vi "CAN_MotorControlandBMS2.vi"() -> ()   [LabVIEW 2018]
uses:
  BMS/OrionBMSClass.lvclass
  <vilib>/Platform/TimedLoop/XDataNode/wakeup.ctl
  <vilib>/Platform/TimedLoop/XDataNode/XDNodeRunTimeDep.lvlib
  <vilib>/Platform/TimedLoop/XDataNode/nitl_modes.ctl
  <vilib>/Platform/TimedLoop/XDataNode/timing_clust.ctl
  <vilib>/platform/TimedLoop/XDataNode/XDataNode.xnode
  Type_Def/Type_Def MotorControlState.ctl
  BMS/MotorControllerClass.lvclass
  Type_Def/TypeDef_MotorData.ctl
  <vilib>/Platform/TimedLoop/XDataNode/loadnilvce.vi
  Type_Def/TypeDef_BMSDatas.ctl
  Type_Def/TypeDef_BMSStatuss.ctl
  Type_Def/Type_Def Actuator Controls.ctl
panel:
  out "BMS2 Freeze":bool
  in  "ReintCAN":bool
  in  "GlobalStop":bool
  in  "Reset BMS Freeze":bool
  in  "stop":bool
  out "Velocity (RPM)":i32
  out "error out":errorcluster
  out "Loop Counter":i32
  out "BMS1 Freeze":bool
  out "stopDriveRes":u32
  out "changeTargetRes":u32
  out "targetTorqueRes":u32
  out "controlWord6Res":i16
  out "startDriveRes":u32
  out "Enum":T1
  in  "error in (no error)":errorcluster
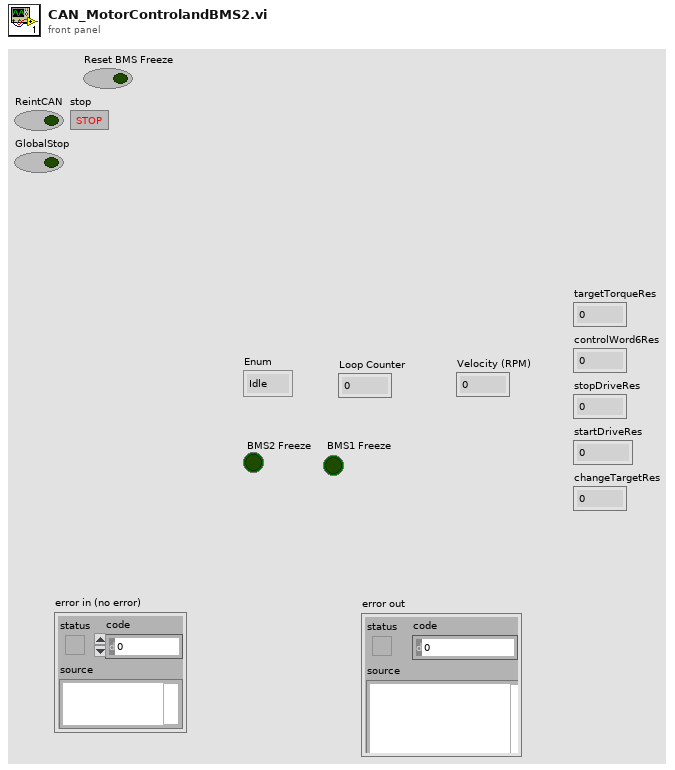
[diagram p1: front panel]
types:
  T1 = typedef "Type_Def MotorControlState.ctl" = enum16{"Idle", "Initialization", "Running", "Termination"}
  T2 = enum32{"1 Mbit/s", "800 kbit/s", "500 kbit/s", "250 kbit/s", "125 kbit/s", "50 kbit/s", "20 kbit/s", "10 kbit/s", ""}
  T3 = typedef "TypeDef_MotorData.ctl" = cluster{" Velocity (RPM)":i32, " MotorTemp(C)":u8, " ControlTemp(C)":u8, " DcLinkVolt(V)":dbl, " ErrorCode":dbl, "IsAlive":bool, "motorStatus":cluster{"isReady":bool, "isOn":bool, "isOperEn":bool, "isFault":bool, "isVoltEn":bool, "targetReached":bool, "isWarning":bool}, "motorControllerState":u16}
  T4 = typedef "XDNodeRunTimeDep.lvlib/timing_clust.ctl" = cluster{"Expected End [f-1]":u64, "Actual End [f-1]":u64, "Finished Late? [f-1]":bool, "Expected End [i-1]":u64, "Actual End [i-1]":u64, "Finished Late? [i-1]":bool, "Expected Start [i]":u64, "Actual Start [i]":u64, "Expected Start [f]":u64, "Actual Start [f]":u64, "Source Name":string, "Structure Name":string, "Period":i64, "Deadline":i64, "Offset":i64, "Start":i64, "Priority":i32, "Timeout":i32, "Mode":T5, "Wakeup Reason":T6, "Error":errorcluster, "Source Type":string, "Secondary Source Type":string, "Global End Time":u64, "Global Start Time":u64, "Frame Duration":u64, "Iteration Duration":u64, "Assigned CPU":i32, "I/O Scan Engine Mode":u32}
  T5 = typedef "XDNodeRunTimeDep.lvlib/nitl_modes.ctl" = enum32{"No Change", "Process missed periods, maintain original phase", "Discard missed periods, maintain original phase", "Process missed periods, ignore original phase", "Discard missed periods, ignore original phase"}
  T6 = typedef "XDNodeRunTimeDep.lvlib/wakeup.ctl" = enum32{"Normal", "Aborted", "Asynchronous wakeup", "Timing source error", "Timed loop error", "Timeout"}
  T7 = typedef "Type_Def Actuator Controls.ctl" = cluster{"Reverse ":bool, "Precharge Ctrl":bool, "Pump Ctrl":bool, "24 VDC Ctr":bool, "Vent Solenoid":bool, "Brake Solenoid":bool, "EMCY  Brake Solenoid":bool, "Digital Out 7B ":bool, "Forward Ctrl":bool, " Contact H2":bool, "Contact L2":bool, "LED RED":bool, "LED GREEN":bool, " Digital Out 7A":bool, " Contact H1":bool, "Contact L1":bool}
  T8 = typedef "TypeDef_BMSDatas.ctl" = cluster{"Pack 1 Max Cell\n Voltage (V)":dbl, "Pack 1 Max Cell\n ID ":dbl, "Pack 1 Min Cell \nVoltage (V)":dbl, "Pack 1 Min Cell \nID ":dbl, "Pack 1 State of Charge  (%)":dbl, "Pack 1 Average Voltage1 (V)":dbl, "Pack 1Voltage Delta (V)":dbl, "Pack 1 Current (A)":dbl, "Pack 1 Voltage (V)":dbl, "Pack 1 Max Resistance (Ohm)":dbl, "Pack 1Min Resistance (Ohm)":dbl, "Pack 1Average Resistance (Ohm)":dbl, "Pack 1Delta Resistance (Ohm)":dbl, "Pack 1 Highest Temperature(C)":dbl, "BmsStatus1":T9, "Pack 2 Max Cell\n Voltage (V) ":dbl, "Pack 2 Max Cell\n ID  ":dbl, "Pack 2 Min Cell \nVoltage (V) ":dbl, "Pack 2 Min Cell \nID  ":dbl, "Pack 2 Average Voltage1 (V)":dbl, "Pack 2 Voltage Delta (V) ":dbl, "Pack 2 Current (A)":dbl, "Pack 2 Voltage (V) ":dbl, "Pack 2 State of Charge  (%) ":dbl, "Pack 2 Max Resistance (Ohm) ":dbl, "Pack 2 Min Resistance (Ohm)":dbl, "Pack 2 Average Resistance (Ohm)":dbl, "Pack 2 Delta Resistance (Ohm) ":dbl, "Pack 2 Highest Temperature(C) ":dbl, "BmsStatus 2":T9}
  T9 = typedef "TypeDef_BMSStatuss.ctl" = cluster{"isFault":bool, "isolationMonitoring":bool}
  T10 = cluster{"error code":dbl, "error register":dbl, "manufacturer specific error field":dbl[]}
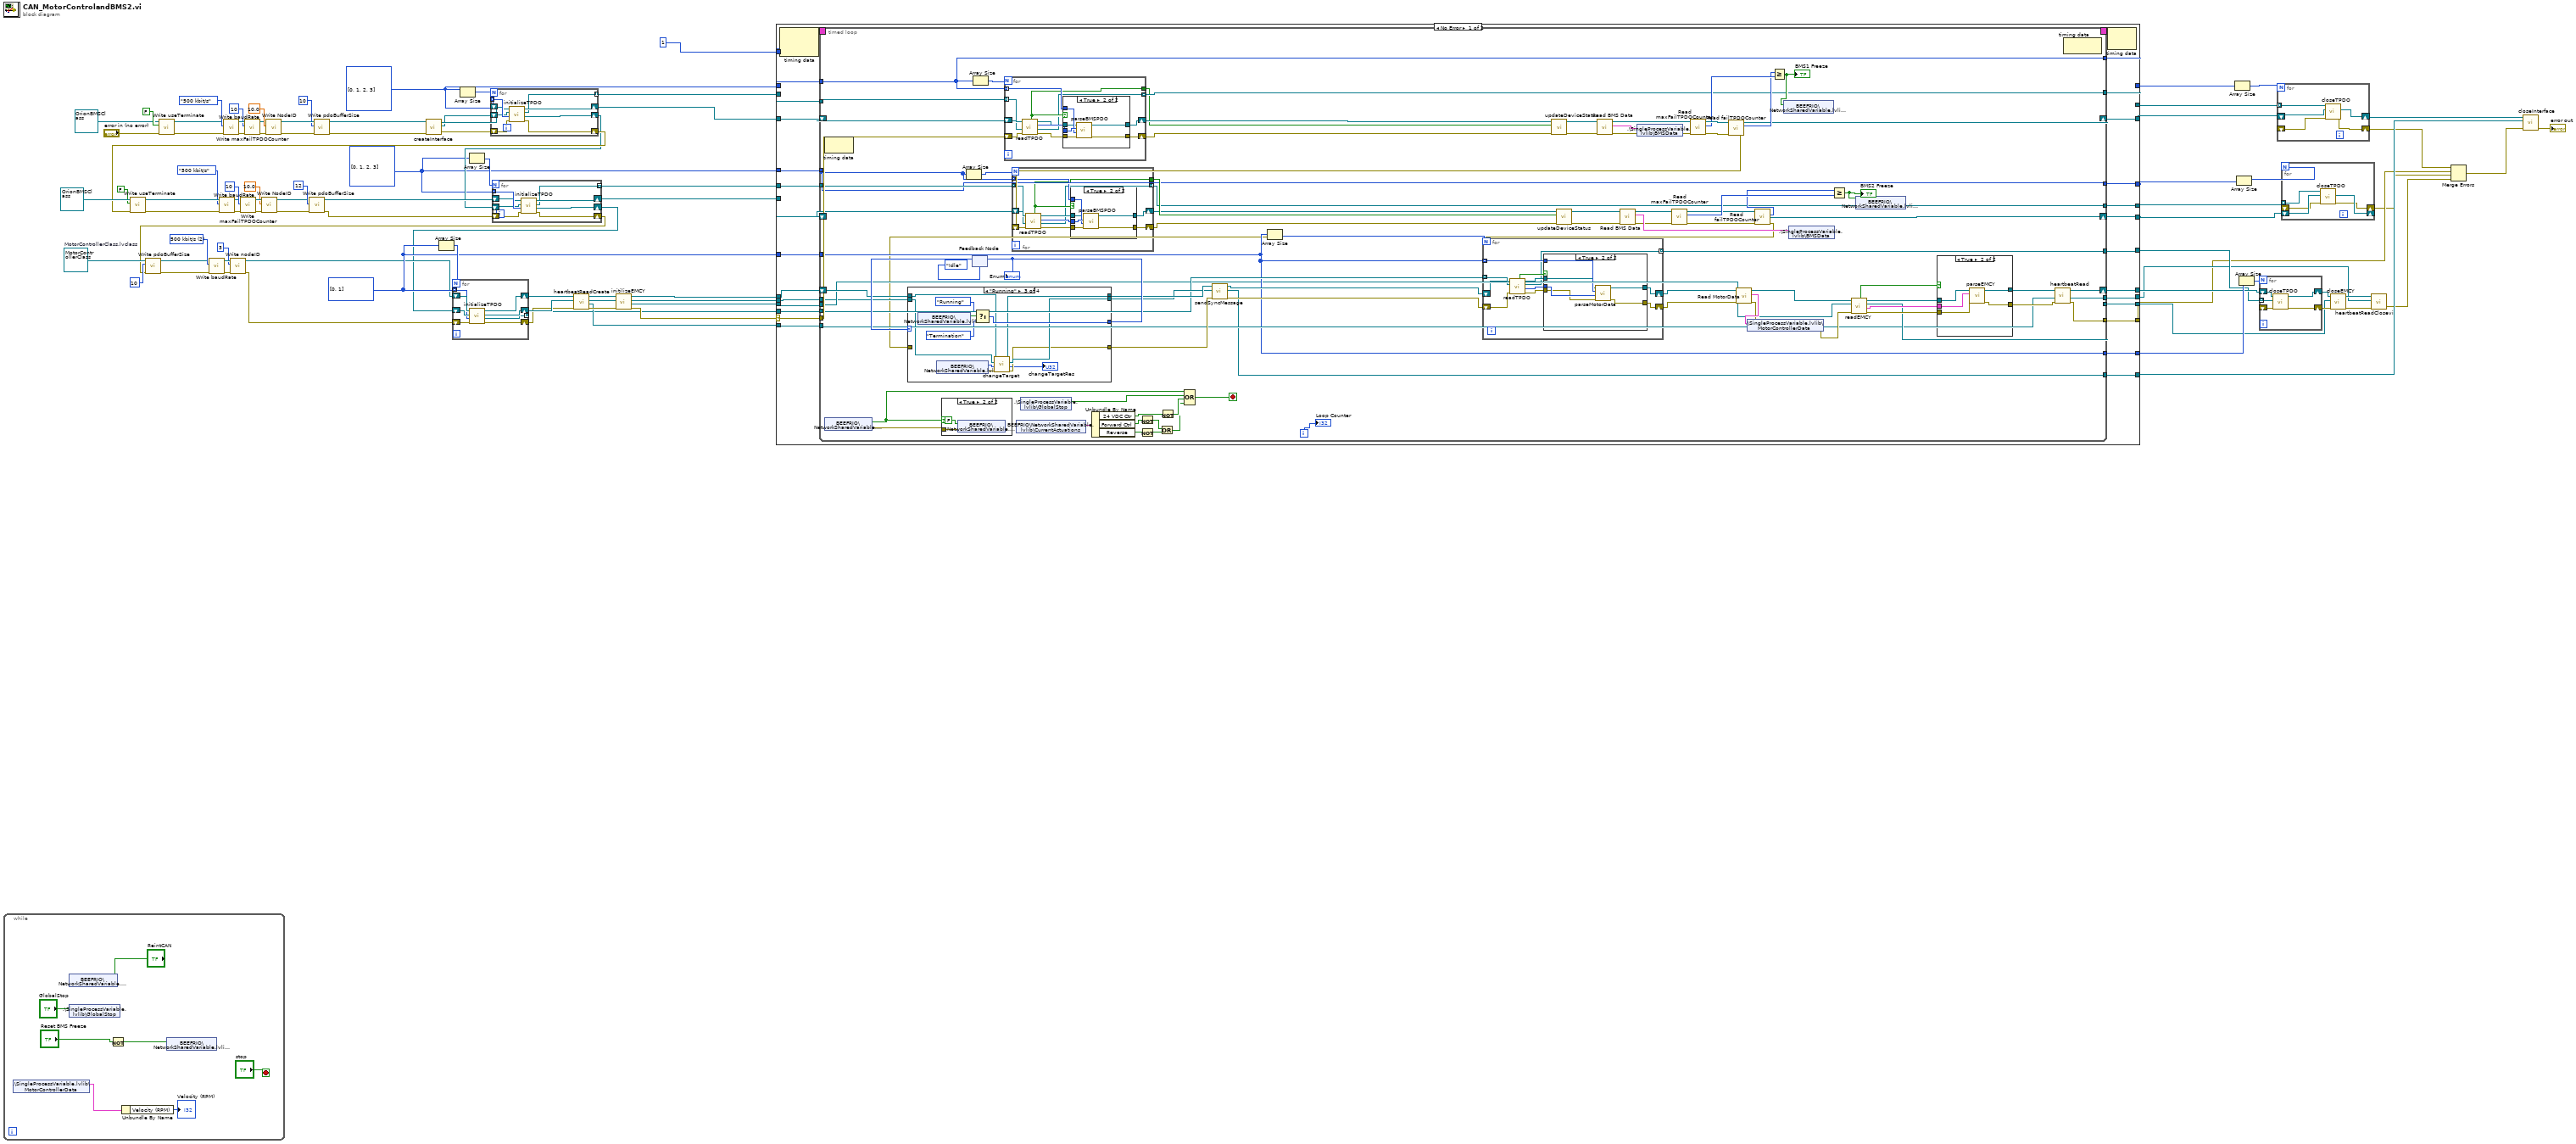
[diagram p0: block diagram]
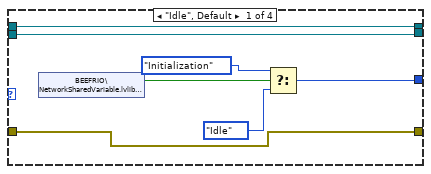
[diagram p6: hidden frame]
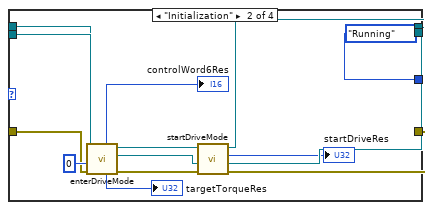
[diagram p7: hidden frame]
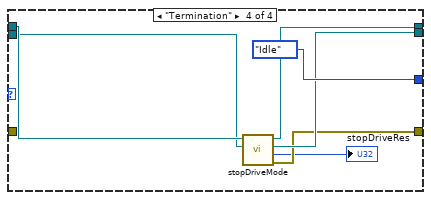
[diagram p8: hidden frame]
diagram:
  w8 = u8[] [0, 1, 2, 3] items=["PDO 1", "PDO 2", "PDO 3", "PDO 4"]
  w46 = u32 2 items=["1 Mbit/s"=0, "800 kbit/s"=1, "500 kbit/s"=2, "250 kbit/s"=3, "125 kbit/s"=4, "50 kbit/s"=6, "20 kbit/s"=7, "10 kbit/s"=8] ("baudRate")
  w78 = u8[] [0, 1] items=["PDO 1", "PDO 2", "PDO 3", "PDO 4"]
  w50 = refnum<class "MotorControllerClass.lvclass"> refnum  # MotorControllerClass.lvclass
  w10 = u8[] [0, 1, 2, 3] items=["PDO 1", "PDO 2", "PDO 3", "PDO 4"]
  n1 = while {
    stop <- "stop" stop-if-true
    n2 = shared-variable ".\\SingleProcessVariable.lvlib\\MotorControllerData"() -> (w101:T3)  [unwired: 1 in, 1 out]
    n3 = shared-variable "BEEFRIO\\NetworkSharedVariable.lvlib\\ReintCAN"("ReintCAN") -> ()  [unwired: 1 in, 1 out]
    n4 = shared-variable ".\\SingleProcessVariable.lvlib\\GlobalStop"("GlobalStop") -> ()  [unwired: 1 in, 1 out]
    n5 = Not(x="Reset BMS Freeze") -> (.not. x?=w103:bool)
    n6 = Unbundle By Name(w101) -> ("Velocity (RPM)"=→"Velocity (RPM)":i32)
    n7 = shared-variable "BEEFRIO\\NetworkSharedVariable.lvlib\\BMSFreeze"(w103) -> ()  [unwired: 1 in, 1 out]
  }
  n8 = call-dynamic "Write useTerminate .vi"("error in (no error)"="error in (no error)", "useTerminate"=FALSE, "OrionBMS in"=refnum<class "OrionBMSClass.lvclass"> refnum ("OrionBMSClass.lvclass")) -> ("error out"=w36:errorcluster, "OrionBMS out"=w37:refnum<class "OrionBMSClass.lvclass">)  [unwired: 7 in]
  n9 = call-dynamic "Write baudRate.vi"("error in (no error)"=w36, "baudRate"=T2."500 kbit/s", "OrionBMSClass in"=w37) -> ("error out"=w42:errorcluster, "OrionBMSClass out"=w43:refnum<class "OrionBMSClass.lvclass">)  [unwired: 7 in]
  n10 = call-dynamic "Write maxFailTPDOCounter.vi"("error in (no error)"=w42, "maxFailTPDOCounter"=u8 10, "OrionBMSClass in"=w43) -> ("error out"=w40:errorcluster, "OrionBMSClass out"=w41:refnum<class "OrionBMSClass.lvclass">)  [unwired: 7 in]
  n11 = call-dynamic "Write NodeID.vi"("error in (no error)"=w40, "NodeID"=10.0, "OrionBMSClass in"=w41) -> ("error out"=w58:errorcluster, "OrionBMSClass out"=w59:refnum<class "OrionBMSClass.lvclass">)  [unwired: 7 in]
  n12 = call-dynamic "Write pdoBufferSize.vi"("error in (no error)"=w58, "pdoBufferSize"=u16 10, "OrionBMSClass in"=w59) -> ("error out"=w56:errorcluster, "OrionBMSClass out"=w57:refnum<class "OrionBMSClass.lvclass">)  [unwired: 7 in]
  n13 = call "createInterface.vi"("error in (no error)"=w56, "OrionBMS in"=w57) -> ("error out"=w95:errorcluster, "interface object out"=w96:refnum<k20>, "OrionBMS out"=w97:refnum<class "OrionBMSClass.lvclass">)  [unwired: 7 in]
  n14 = Array Size(array=w78) -> (size(s)=w89:i32)
  n15 = Array Size(array=w10) -> (size(s)=w11:i32)
  n16 = Array Size(array=w8) -> (size(s)=w9:i32)
  n17 = for {
    N: w11 -> [_]
    tunnel: w10 -> [w114] mode=indexing
    shift-right: [w110] -> w94
    shift-left: w97 -> [w113]
    tunnel: [w107] -> w93 mode=indexing
    shift-right: [w109] -> w12
    shift-left: w96 -> [w112]
    shift-right: [w108] -> w16
    shift-left: w95 -> [w111]
    n18 = call "initializeTPDO.vi"("error in (no error)"=w111, "PDO channel"=w114, "interface object in"=w112, "OrionBMS in"=w113) -> ("error out"=w108:errorcluster, "interface object out"=w109:refnum<k20>, "TPDO object out"=w107:refnum<k20>, "OrionBMS out"=w110:refnum<class "OrionBMSClass.lvclass">)  [unwired: 2 in]
  }
  n19 = call-dynamic "Write useTerminate .vi"("error in (no error)"=w16, "useTerminate"=FALSE, "OrionBMS in"=refnum<class "OrionBMSClass.lvclass"> refnum ("OrionBMSClass.lvclass")) -> ("error out"=w32:errorcluster, "OrionBMS out"=w31:refnum<class "OrionBMSClass.lvclass">)  [unwired: 7 in]
  n20 = call-dynamic "Write baudRate.vi"("error in (no error)"=w32, "baudRate"=T2."500 kbit/s", "OrionBMSClass in"=w31) -> ("error out"=w27:errorcluster, "OrionBMSClass out"=w26:refnum<class "OrionBMSClass.lvclass">)  [unwired: 7 in]
  n21 = call-dynamic "Write maxFailTPDOCounter.vi"("error in (no error)"=w27, "maxFailTPDOCounter"=u8 10, "OrionBMSClass in"=w26) -> ("error out"=w29:errorcluster, "OrionBMSClass out"=w28:refnum<class "OrionBMSClass.lvclass">)  [unwired: 7 in]
  n22 = call-dynamic "Write NodeID.vi"("error in (no error)"=w29, "NodeID"=10.0, "OrionBMSClass in"=w28) -> ("error out"=w22:errorcluster, "OrionBMSClass out"=w21:refnum<class "OrionBMSClass.lvclass">)  [unwired: 7 in]
  n23 = call-dynamic "Write pdoBufferSize.vi"("error in (no error)"=w22, "pdoBufferSize"=u16 12, "OrionBMSClass in"=w21) -> ("error out"=w19:errorcluster, "OrionBMSClass out"=w18:refnum<class "OrionBMSClass.lvclass">)  [unwired: 7 in]
  n24 = for {
    N: w9 -> [_]
    tunnel: w8 -> [w122] mode=indexing
    shift-right: [w118] -> w13
    shift-left: w18 -> [w121]
    tunnel: [w115] -> w14 mode=indexing
    shift-right: [w117] -> w1
    shift-left: w12 -> [w120]
    shift-right: [w116] -> w15
    shift-left: w19 -> [w119]
    n25 = call "initializeTPDO.vi"("error in (no error)"=w119, "PDO channel"=w122, "interface object in"=w120, "OrionBMS in"=w121) -> ("error out"=w116:errorcluster, "interface object out"=w117:refnum<k20>, "TPDO object out"=w115:refnum<k20>, "OrionBMS out"=w118:refnum<class "OrionBMSClass.lvclass">)  [unwired: 2 in]
  }
  n26 = call-dynamic "Write pdoBufferSize.vi"("error in (no error)"=w15, "pdoBufferSize"=u16 10, "MotorControllerClass in"=w50) -> ("error out"=w33:errorcluster, "MotorControllerClass out"=w34:refnum<class "MotorControllerClass.lvclass">)  [unwired: 7 in]
  n27 = call-dynamic "Write baudRate.vi"("error in (no error)"=w33, "baudRate"=w46, "MotorControllerClass in"=w34) -> ("error out"=w49:errorcluster, "MotorControllerClass out"=w52:refnum<class "MotorControllerClass.lvclass">)  [unwired: 7 in]
  n28 = call-dynamic "Write nodeID.vi"("error in (no error)"=w49, "nodeID"=u8 3, "MotorControllerClass in"=w52) -> ("error out"=w48:errorcluster, "MotorControllerClass out"=w51:refnum<class "MotorControllerClass.lvclass">)  [unwired: 7 in]
  n29 = for {
    N: w89 -> [_]
    tunnel: w78 -> [w128] mode=indexing
    tunnel: [w125] -> w77 mode=indexing
    shift-right: [w127] -> w88
    shift-left: w51 -> [w130]
    shift-right: [w126] -> w87
    shift-left: w1 -> [w129]
    shift-right: [w124] -> w86
    shift-left: w48 -> [w123]
    n30 = call "initializeTPDO.vi"("error in (no error)"=w123, "PDO channel"=w128, "interface object in"=w129, "MotorControllerClass in"=w130) -> ("error out"=w124:errorcluster, "TPDO object out"=w125:refnum<k20>, "interface object out"=w126:refnum<k20>, "MotorControllerClass out"=w127:refnum<class "MotorControllerClass.lvclass">)  [unwired: 4 in]
  }
  n31 = call "heartbeatReadCreate.vi"("error in (no error)"=w86, "interface object in"=w87, "MotorControllerClass in"=w88) -> ("error out"=w83:errorcluster, "heartbeat object out"=w82:refnum<k20>, "interface object out"=w84:refnum<k20>, "MotorControllerClass out"=w85:refnum<class "MotorControllerClass.lvclass">)  [unwired: 5 in]
  n32 = call "initilizeEMCY.vi"("error in (no error)"=w83, "interface object in"=w84, "MotorControllerClass in"=w85) -> ("error out"=w81:errorcluster, "emergency object out"=w35:refnum<k20>, "interface object out"=w79:refnum<k20>, "MotorControllerClass out"=w80:refnum<class "MotorControllerClass.lvclass">)  [unwired: 5 in]
  n33 = case shown="No Error" w81 {
    selector: w81 -> [w141 w369]
    tunnel: w10 -> [w157 w372]
    tunnel: w94 -> [w156 w371]
    tunnel: w93 -> [w155 w364]
    tunnel: [w132 w372] -> w75
    tunnel: [w151 w364] -> w38
    tunnel: w82 -> [w154 w366]
    tunnel: w80 -> [w142 w367]
    tunnel: w79 -> [w140 w365]
    tunnel: w78 -> [w153 w370]
    tunnel: w77 -> [w152 w368]
    tunnel: [w131 w371] -> w74
    tunnel: [w150 w366] -> w64
    tunnel: [w144 w363] -> w67
    tunnel: [w149 w369] -> w61
    tunnel: [w148 w370] -> w73
    tunnel: [w147 w367] -> w71
    tunnel: [w145 w368] -> w70
    tunnel: [w146 w365] -> w63
    tunnel: i64 1 ("Period") -> [w143 _]
    tunnel: w35 -> [w139 w363]
    tunnel: w14 -> [w138 w361]
    tunnel: w13 -> [w136 w360]
    tunnel: w8 -> [w137 w362]
    tunnel: [w135 w360] -> w5
    tunnel: [w134 w361] -> w6
    tunnel: [w133 w362] -> w4
    frame No Error {
      n34 = node-c288(w143) -> (w159:T4)  [unwired: 1 in]
      n35 = timed-loop {
        timing: w159 -> [_]
        timing-out: [_] -> w158
        tunnel: w157 -> [w230]
        tunnel: w155 -> [w244]
        tunnel: [w230] -> w132
        tunnel: [w229] -> w151
        tunnel: w154 -> [w204]
        tunnel: w153 -> [w201]
        tunnel: w152 -> [w220]
        tunnel: [w207] -> w144
        tunnel: [w203] -> w149
        tunnel: [w202] -> w150
        tunnel: [w201] -> w148
        shift-right: [w200] -> w147
        shift-left: w142 -> [w225]
        tunnel: [w199] -> w145
        tunnel: [w198] -> w146
        tunnel: w139 -> [w187]
        tunnel: w141 -> [w226]
        tunnel: w140 -> [w185]
        shift-right: [w184] -> w131
        shift-left: w156 -> [w245]
        tunnel: w138 -> [w182]
        tunnel: w137 -> [w167]
        tunnel: [w167] -> w133
        tunnel: [w166] -> w134
        shift-right: [w165] -> w135
        shift-left: w136 -> [w163]
        i -> [w247]
        stop <- w161 stop-if-true
        n36 = node-c288() -> ()  [unwired: 1 in, 1 out]
        n37 = shared-variable "BEEFRIO\\NetworkSharedVariable.lvlib\\ReintCAN"() -> (w160:bool, error out=w193:errorcluster)  [unwired: 1 in]
        n38 = case shown="True" w160 {
          tunnel: w193 -> [_ w268]
          frame False {
          }
          frame True {
            n39 = shared-variable "BEEFRIO\\NetworkSharedVariable.lvlib\\ReintCAN"(FALSE ("ReintCAN"), error in=w268) -> ()  [unwired: 1 out]
          }
        }
        n40 = Array Size(array=w167) -> (size(s)=w183:i32)
        n41 = feedback #1(Type_Def_MotorControlState."Idle" ("Enum")) -> (w227:T1)
        n42 = Array Size(array=w230) -> (size(s)=w246:i32)
        n43 = for {
          N: w246 -> [_]
          tunnel: w244 -> [w344] mode=indexing
          tunnel: w230 -> [w341] mode=indexing
          tunnel: [w339] -> w162
          shift-right: [w338] -> w243
          shift-left: w245 -> [w345]
          shift-right: [w336] -> w242
          shift-left: w226 -> [w337]
          tunnel: [w335] -> w229 mode=indexing
          n44 = call "readTPDO.vi"("OrionBMS.lvclass"=w345, "TPDO object in"=w344, "error in (no error)"=w337) -> ("new data?"=w339:bool, "OrionBMS.lvclass"=w340:refnum<class "OrionBMSClass.lvclass">, "TPDO data"=w343:u8[], "TPDO object out"=w335:refnum<k20>, "error out"=w342:errorcluster)  [unwired: 3 in]
          n45 = case shown="True" w339 {
            tunnel: w343 -> [_ w353]
            tunnel: w342 -> [w346 w352]
            tunnel: w341 -> [_ w351]
            tunnel: w340 -> [w347 w350]
            tunnel: [w347 w349] -> w338
            tunnel: [w346 w348] -> w336
            frame False {
            }
            frame True {
              n46 = call "parseBMSPDO.vi"("error in (no error)"=w352, "PDO channel"=w351, "TPDO data"=w353, "OrionBMS in"=w350) -> ("error out"=w348:errorcluster, "OrionBMS out"=w349:refnum<class "OrionBMSClass.lvclass">)  [unwired: 6 in]
            }
          }
        }
        n47 = shared-variable "BEEFRIO\\NetworkSharedVariable.lvlib\\CurrentActuations"() -> (w197:T7)  [unwired: 1 in, 1 out]
        n48 = shared-variable ".\\SingleProcessVariable.lvlib\\GlobalStop"() -> (w194:bool)  [unwired: 1 in, 1 out]
        n49 = Unbundle By Name(w197) -> ("24 VDC Ctr"=w196:bool, "Forward Ctrl"=w192:bool, "Reverse"=w191:bool)
        n50 = Not(x=w192) -> (.not. x?=w190:bool)
        n51 = Not(x=w191) -> (.not. x?=w189:bool)
        n52 = Or(x=w190, y=w189) -> (x .or. y?=w188:bool)
        n53 = Not(x=w196) -> (.not. x?=w195:bool)
        n54 = Compound Arithmetic op=OR(w160, w194, w195, w188) -> (w161:bool)
        n55 = Array Size(array=w201) -> (size(s)=w221:i32)
        n56 = call "updateDeviceStatus.vi"("OrionBMS in"=w243, "isNewData"=w162, "error in (no error)"=w242) -> ("OrionBMS out"=w241:refnum<class "OrionBMSClass.lvclass">, "error out"=w240:errorcluster)  [unwired: 6 in]
        n57 = call-dynamic "Read BMS Data.vi"("error in (no error)"=w240, "OrionBMS in"=w241) -> ("error out"=w238:errorcluster, "BMS Data"=w239:T8, "OrionBMS out"=w235:refnum<class "OrionBMSClass.lvclass">)  [unwired: 7 in]
        n58 = shared-variable ".\\SingleProcessVariable.lvlib\\BMSData"(w239, error in=w238) -> (error out=w237:errorcluster)
        n59 = call-dynamic "Read maxFailTPDOCounter.vi"("error in (no error)"=w237, "OrionBMS in"=w235) -> ("error out"=w236:errorcluster, "maxFailTPDOCounter"=w233:u8, "OrionBMS out"=w234:refnum<class "OrionBMSClass.lvclass">)  [unwired: 7 in]
        n60 = call-dynamic "Read failTPDOCounter.vi"("error in (no error)"=w236, "OrionBMS in"=w234) -> ("error out"=w181:errorcluster, "failTPDOCounter"=w232:u8, "OrionBMS out"=w184:refnum<class "OrionBMSClass.lvclass">)  [unwired: 7 in]
        n61 = for {
          N: w183 -> [_]
          tunnel: w182 -> [w257] mode=indexing
          tunnel: w167 -> [w254] mode=indexing
          tunnel: [w252] -> w175
          shift-right: [w251] -> w174
          shift-left: w163 -> [w258]
          shift-right: [w249] -> w172
          shift-left: w181 -> [w250]
          tunnel: [w248] -> w166 mode=indexing
          n62 = call "readTPDO.vi"("OrionBMS.lvclass"=w258, "TPDO object in"=w257, "error in (no error)"=w250) -> ("new data?"=w252:bool, "OrionBMS.lvclass"=w253:refnum<class "OrionBMSClass.lvclass">, "TPDO data"=w256:u8[], "TPDO object out"=w248:refnum<k20>, "error out"=w255:errorcluster)  [unwired: 3 in]
          n63 = case shown="True" w252 {
            tunnel: w256 -> [_ w266]
            tunnel: w255 -> [w259 w265]
            tunnel: w254 -> [_ w264]
            tunnel: w253 -> [w260 w263]
            tunnel: [w260 w262] -> w251
            tunnel: [w259 w261] -> w249
            frame False {
            }
            frame True {
              n64 = call "parseBMSPDO.vi"("error in (no error)"=w265, "PDO channel"=w264, "TPDO data"=w266, "OrionBMS in"=w263) -> ("error out"=w261:errorcluster, "OrionBMS out"=w262:refnum<class "OrionBMSClass.lvclass">)  [unwired: 6 in]
            }
          }
        }
        n65 = call "updateDeviceStatus.vi"("OrionBMS in"=w174, "isNewData"=w175, "error in (no error)"=w172) -> ("OrionBMS out"=w173:refnum<class "OrionBMSClass.lvclass">, "error out"=w171:errorcluster)  [unwired: 6 in]
        n66 = call-dynamic "Read BMS Data.vi"("error in (no error)"=w171, "OrionBMS in"=w173) -> ("error out"=w170:errorcluster, "BMS Data"=w176:T8, "OrionBMS out"=w177:refnum<class "OrionBMSClass.lvclass">)  [unwired: 7 in]
        n67 = call-dynamic "Read maxFailTPDOCounter.vi"("error in (no error)"=w170, "OrionBMS in"=w177) -> ("error out"=w169:errorcluster, "maxFailTPDOCounter"=w179:u8, "OrionBMS out"=w178:refnum<class "OrionBMSClass.lvclass">)  [unwired: 7 in]
        n68 = call-dynamic "Read failTPDOCounter.vi"("error in (no error)"=w169, "OrionBMS in"=w178) -> ("error out"=w164:errorcluster, "failTPDOCounter"=w168:u8, "OrionBMS out"=w165:refnum<class "OrionBMSClass.lvclass">)  [unwired: 7 in]
        n69 = case shown="\"Running\"" w227 {
          tunnel: [w300 Type_Def_MotorControlState."Running" ("Enum") w324 Type_Def_MotorControlState."Idle" ("Enum")] -> w228
          tunnel: [w299 w305 w319 w331] -> w224
          tunnel: w225 -> [w299 w311 w322 w333]
          tunnel: [w298 w306 w318 w330] -> w223
          tunnel: w185 -> [w298 w312 w321 w332]
          tunnel: [w295 w303 w317 w329] -> w222
          tunnel: w164 -> [w295 w302 _ _]
          frame "Idle", Default {
            n70 = shared-variable "BEEFRIO\\NetworkSharedVariable.lvlib\\driveEnable"() -> (w301:bool)  [unwired: 1 in, 1 out]
            n71 = Select(t=Type_Def_MotorControlState."Initialization" ("Enum"), s=w301, f=Type_Def_MotorControlState."Idle" ("Enum")) -> (s? t:f=w300:T1)
          }
          frame "Initialization" {
            n72 = call "enterDriveMode.vi"("error in (no error)"=w302, "targetNumber"=i16 0, "interface object in"=w312, "MotorControllerClass in"=w311) -> ("error out"=w307:errorcluster, "interface object out"=w308:refnum<k20>, "MotorControllerClass out"=w309:refnum<class "MotorControllerClass.lvclass">, "targetTorqueRes"=→"targetTorqueRes":u32, "controlWord6Res"=→"controlWord6Res":i16)  [unwired: 3 in]
            n73 = call "startDriveMode.vi"("error in (no error)"=w307, "interface object in"=w308, "MotorControllerClass in"=w309) -> ("error out"=w303:errorcluster, "interface object out"=w306:refnum<k20>, "startDriveRes"=→"startDriveRes":u32, "MotorControllerClass out"=w305:refnum<class "MotorControllerClass.lvclass">)  [unwired: 5 in]
          }
          frame "Running" {
            n74 = shared-variable "BEEFRIO\\NetworkSharedVariable.lvlib\\driveEnable"() -> (w327:bool)  [unwired: 1 in, 1 out]
            n75 = shared-variable "BEEFRIO\\NetworkSharedVariable.lvlib\\driveTarget"() -> (w323:i16, error out=w320:errorcluster)  [unwired: 1 in]
            n76 = Select(t=Type_Def_MotorControlState."Running" ("Enum"), s=w327, f=Type_Def_MotorControlState."Termination" ("Enum")) -> (s? t:f=w324:T1)
            n77 = call "changeTarget.vi"("error in (no error)"=w320, "targetNumber"=w323, "interface object in"=w321, "MotorControllerClass in"=w322) -> ("error out"=w317:errorcluster, "changeTargetRes"=→"changeTargetRes":u32, "interface object out"=w318:refnum<k20>, "MotorControllerClass out"=w319:refnum<class "MotorControllerClass.lvclass">)  [unwired: 4 in]
          }
          frame "Termination" {
            n78 = call "stopDriveMode.vi"("interface object in"=w332, "MotorControllerClass in"=w333) -> ("error out"=w329:errorcluster, "stopDriveRes"=→"stopDriveRes":u32, "interface object out"=w330:refnum<k20>, "MotorControllerClass out"=w331:refnum<class "MotorControllerClass.lvclass">)  [unwired: 6 in]
          }
        }
        "Enum" <- w228
        n79 = feedback-in #1(w228) -> ()
        n80 = call "sendSyncMessage.vi"("error in (no error)"=w222, "interface object in"=w223, "MotorControllerClass in"=w224) -> ("error out"=w218:errorcluster, "interface object out"=w198:refnum<k20>, "MotorControllerClass out"=w219:refnum<class "MotorControllerClass.lvclass">)  [unwired: 6 in]
        n81 = for {
          N: w221 -> [_]
          tunnel: w201 -> [w279] mode=indexing
          tunnel: w220 -> [w286] mode=indexing
          shift-right: [w278] -> w217
          shift-left: w219 -> [w285]
          shift-right: [w277] -> w216
          shift-left: w218 -> [w284]
          tunnel: [w276] -> w199 mode=indexing
          n82 = call "readTPDO.vi"("error in (no error)"=w284, "TPDO object in"=w286, "MotorControllerClass in"=w285) -> ("error out"=w281:errorcluster, "TPDO data"=w282:u8[], "TPDO object out"=w276:refnum<k20>, "MotorControllerClass out"=w280:refnum<class "MotorControllerClass.lvclass">, "new data?"=w283:bool)  [unwired: 4 in]
          n83 = case shown="True" w283 {
            tunnel: w282 -> [_ w292]
            tunnel: w281 -> [w287 w291]
            tunnel: w280 -> [w288 w293]
            tunnel: w279 -> [_ w294]
            tunnel: [w288 w290] -> w278
            tunnel: [w287 w289] -> w277
            frame False {
            }
            frame True {
              n84 = call "parseMotorData.vi"("error in (no error)"=w291, "TPDO data"=w292, "PDO channel"=w294, "MotorControllerClass in"=w293) -> ("error out"=w289:errorcluster, "MotorControllerClass out"=w290:refnum<class "MotorControllerClass.lvclass">)  [unwired: 6 in]
            }
          }
        }
        n85 = call-dynamic "Read MotorData.vi"("error in (no error)"=w216, "MotorControllerClass in"=w217) -> ("error out"=w214:errorcluster, "MotorData"=w215:T3, "MotorControllerClass out"=w213:refnum<class "MotorControllerClass.lvclass">)  [unwired: 7 in]
        n86 = shared-variable ".\\SingleProcessVariable.lvlib\\MotorControllerData"(w215, error in=w214) -> (error out=w212:errorcluster)
        n87 = Greater Or Equal?(x=w232, y=w233) -> (x >= y?=w231:bool)
        "BMS1 Freeze" <- w231
        n88 = shared-variable "BEEFRIO\\NetworkSharedVariable.lvlib\\BMSFreeze"(w231) -> ()  [unwired: 1 in, 1 out]
        n89 = shared-variable ".\\SingleProcessVariable.lvlib\\BMSData"(w176) -> ()  [unwired: 1 in, 1 out]
        n90 = Greater Or Equal?(x=w168, y=w179) -> (x >= y?=w180:bool)
        "BMS2 Freeze" <- w180
        n91 = call "readEMCY.vi"("error in (no error)"=w212, "emergency object in"=w187, "MotorControllerClass in"=w213) -> ("error out"=w208:errorcluster, "emergency message"=w209:T10, "emergency object out"=w207:refnum<k20>, "MotorControllerClass out"=w210:refnum<class "MotorControllerClass.lvclass">, "isNewMessage"=w211:bool)  [unwired: 4 in]
        n92 = shared-variable "BEEFRIO\\NetworkSharedVariable.lvlib\\BMSFreeze"(w180) -> ()  [unwired: 1 in, 1 out]
        n93 = case shown="True" w211 {
          tunnel: w210 -> [w270 w275]
          tunnel: w209 -> [_ w274]
          tunnel: w208 -> [w269 w273]
          tunnel: [w270 w272] -> w206
          tunnel: [w269 w271] -> w205
          frame False {
          }
          frame True {
            n94 = call "parseEMCY.vi"("error in (no error)"=w273, "emergency message"=w274, "MotorControllerClass in"=w275) -> ("error out"=w271:errorcluster, "MotorControllerClass out"=w272:refnum<class "MotorControllerClass.lvclass">)  [unwired: 7 in]
          }
        }
        n95 = call "heartbeatRead.vi"("error in (no error)"=w205, "heartbeat object in"=w204, "MotorControllerClass in"=w206) -> ("error out"=w203:errorcluster, "heartbeat object out"=w202:refnum<k20>, "MotorControllerClass out"=w200:refnum<class "MotorControllerClass.lvclass">)  [unwired: 6 in]
        n96 = node-c288() -> ()  [unwired: 1 in, 1 out]
        "Loop Counter" <- w247
      }
      n97 = node-c288(w158) -> ()  [unwired: 1 out]
    }
    frame Error {
    }
  }
  n98 = Array Size(array=w75) -> (size(s)=w92:i32)
  n99 = Array Size(array=w4) -> (size(s)=w7:i32)
  n100 = Array Size(array=w73) -> (size(s)=w72:i32)
  n101 = for {
    N: w72 -> [_]
    tunnel: w70 -> [w376] mode=indexing
    shift-right: [w374] -> w68
    shift-left: _ -> [w375]
    shift-right: [w373] -> w69
    shift-left: w71 -> [w377]
    n102 = call "closeTPDO.vi"("error in (no error)"=w375, "TPDO object in"=w376, "MotorControllerClass in"=w377) -> ("error out"=w374:errorcluster, "MotorControllerClass out"=w373:refnum<class "MotorControllerClass.lvclass">)  [unwired: 7 in]
  }
  n103 = for {
    N: w92 -> [_]
    tunnel: w38 -> [w381] mode=indexing
    shift-right: [w380] -> w91
    shift-left: w74 -> [w378]
    shift-right: [w379] -> w62
    shift-left: _ -> [w382]
    n104 = call "closeTPDO.vi"("error in (no error)"=w382, "OrionBMSClass in"=w378, "TPDO object in"=w381) -> ("error in (no error) 2"=w379:errorcluster, "OrionBMSClass out"=w380:refnum<class "OrionBMSClass.lvclass">)  [unwired: 5 in]
  }
  n105 = for {
    N: w7 -> [_]
    tunnel: w6 -> [w385] mode=indexing
    shift-right: [w384] -> _
    shift-left: w5 -> [w387]
    shift-right: [w383] -> w3
    shift-left: _ -> [w386]
    n106 = call "closeTPDO.vi"("error in (no error)"=w386, "OrionBMSClass in"=w387, "TPDO object in"=w385) -> ("error in (no error) 2"=w383:errorcluster, "OrionBMSClass out"=w384:refnum<class "OrionBMSClass.lvclass">)  [unwired: 5 in]
  }
  n107 = call "closeEMCY.vi"("error in (no error)"=w68, "emergency object in"=w67, "MotorControllerClass in"=w69) -> ("error out"=w65:errorcluster, "MotorControllerClass out"=w66:refnum<class "MotorControllerClass.lvclass">)  [unwired: 7 in]
  n108 = call "heartbeatReadClosevi.vi"("error in (no error)"=w65, "heartbeat object in"=w64, "MotorControllerClass in"=w66) -> ("error out"=w2:errorcluster)  [unwired: 7 in, 1 out]
  n109 = Merge Errors(w62, w61, w3, w2) -> (w76:errorcluster)
  n110 = call "closeInterface.vi"("error in (no error)"=w76, "interface object in"=w63, "OrionBMS.lvclass"=w91) -> ("error out"=→"error out":errorcluster)  [unwired: 5 in, 1 out]
